vi "Decode.vi"(8 "error in (no error)":errorcluster, 10 "Base64 String":string, 11 "Serializer.Base64 in":refnum<class "Serializer.Base64.lvclass">) -> (0 "error out":errorcluster, 2 "decoded string":string, 3 "Serializer.Base64 out":refnum<class "Serializer.Base64.lvclass">)   [LabVIEW 2017, in "Serializer.Base64.lvclass"]
uses:
  Serializer.Base64.lvclass
  Serializer.Base64.lvclass/Serializer.Base64.ctl
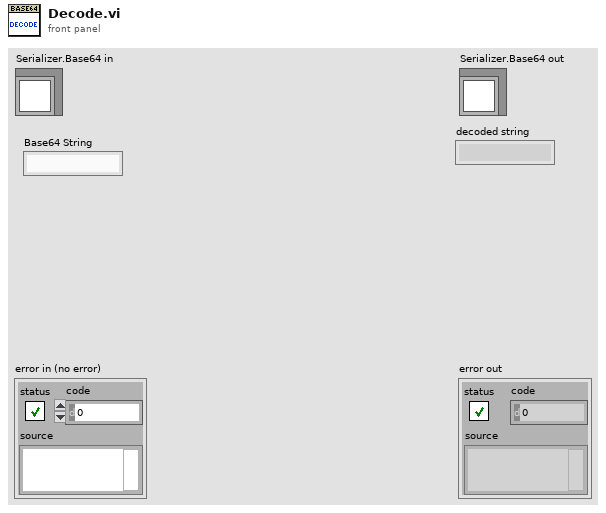
[diagram p1: front panel]
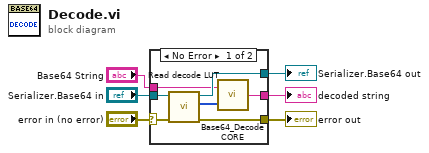
[diagram p0: block diagram]
diagram:
  n1 = case shown="No Error" "error in (no error)" {
    selector: "error in (no error)" -> [w8 w15]
    tunnel: [w7 w15] -> w5
    tunnel: [w12 w14] -> w3
    tunnel: "Serializer.Base64 in" -> [w13 w14]
    tunnel: "Base64 String" -> [w10 _]
    tunnel: [w9 _] -> w1
    frame No Error {
      n2 = call "Read decode LUT.vi"("error in (no error)"=w8, "Serializer.Base64 in"=w13) -> ("error out"=w7:errorcluster, "decode LUT"=w11:u32[], "Serializer.Base64 out"=w12:refnum<class "Serializer.Base64.lvclass">)  [unwired: 7 in]
      n3 = call "Base64_Decode CORE.vi"("Decode LUT"=w11, "Base64 String"=w10) -> ("string"=w9:string)
    }
    frame Error {
    }
  }
  "error out" <- w5
  "Serializer.Base64 out" <- w3
  "decoded string" <- w1
